vi "超标留样启动流程.vi"   [LabVIEW 2016, in "超标留样集成.lvlib" / "德润DR803L超标留样.lvlib"]
types:
  T1 = enum16{"open", "read", "write", "write single", "close"}
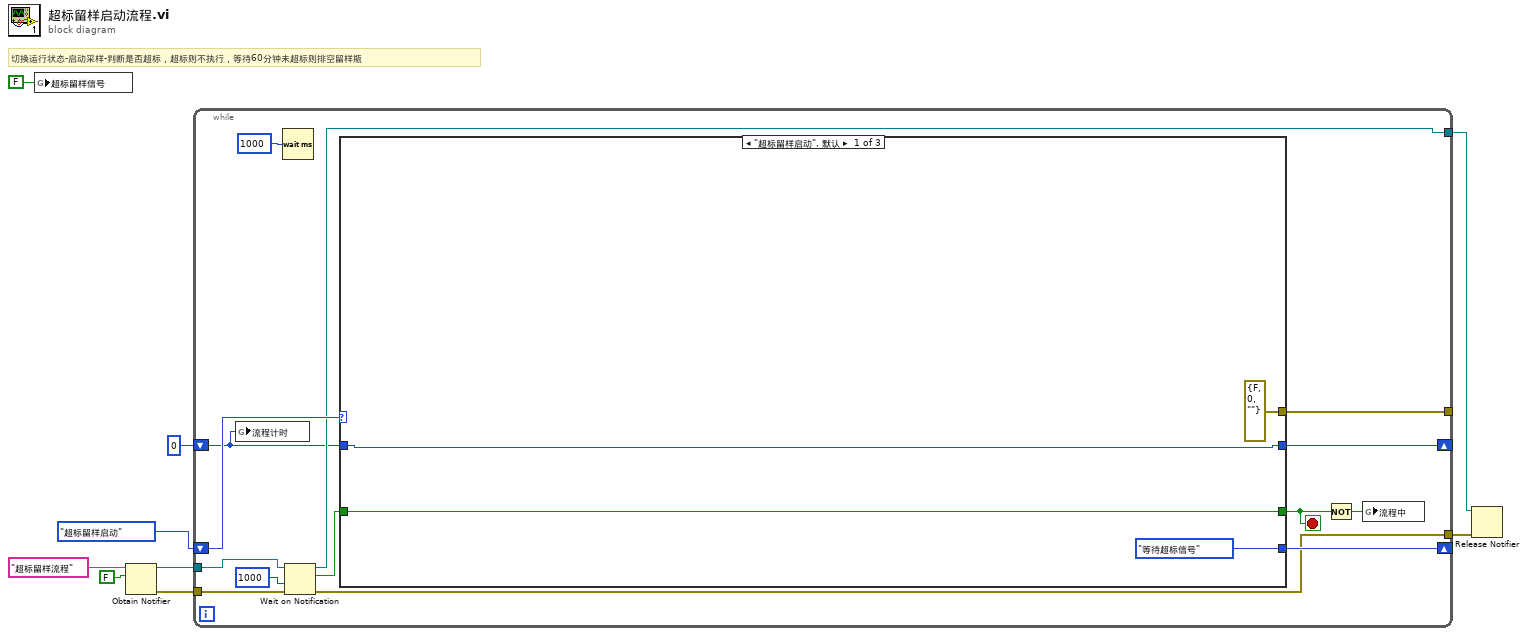
[diagram p0: block diagram]
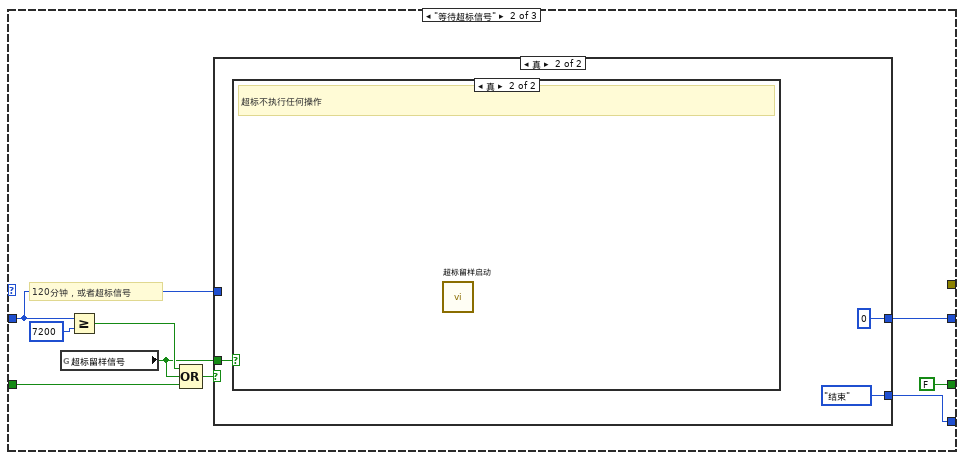
[diagram p2: hidden frame]
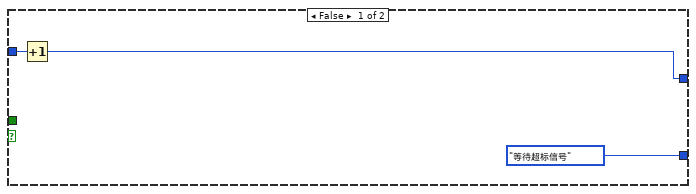
[diagram p3: hidden frame]
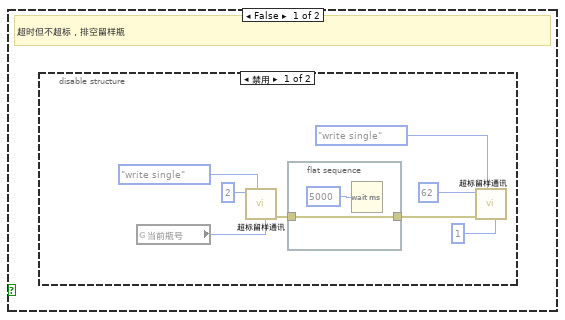
[diagram p4: hidden frame]
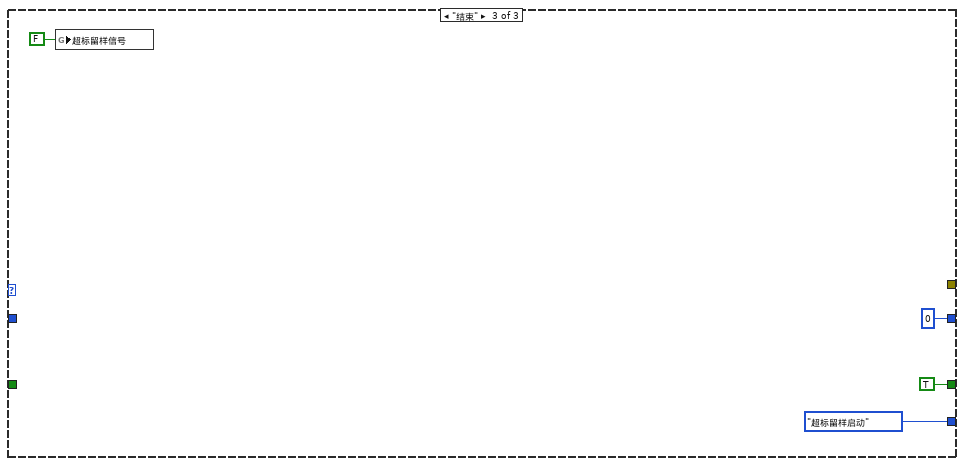
[diagram p6: hidden frame]
diagram:
  # "切换运行状态-启动采样-判断是否超标，超标则不执行，等待60分钟未超标则排空留样瓶"
  n1 = global write "串口参数断电保存全局变量.vi" "超标留样信号"(FALSE ("采样完成")) -> ()
  n2 = Obtain Notifier(name (unnamed)="超标留样流程" ("名称（未命名）"), notification data type=FALSE ("采样完成")) -> (notifier out=w5:refnum<notifier>, error out=w4:errorcluster)  [unwired: 2 in, 1 out]
  n3 = while {
    shift-right: [w17] -> _
    shift-left: enum16{"超标留样启动", "等待超标信号", "结束"}."超标留样启动" -> [w23]
    shift-right: [w21] -> _
    shift-left: 0 -> [w10]
    tunnel: w5 -> [w20]
    tunnel: w4 -> [w19]
    tunnel: [w15] -> _
    tunnel: [w12] -> w2
    tunnel: [w11] -> w1
    stop <- w13 stop-if-true
    n4 = global write "串口参数断电保存全局变量.vi" "流程计时"(w10) -> ()
    n5 = Wait (ms)(milliseconds to wait=u32 1000 ("等待时间（毫秒）")) -> ()  [unwired: 1 out]
    n6 = Wait on Notification(notifier=w20, timeout in ms (-1)=1000 ("超时毫秒(-1)"), error in (no error)=w19) -> (notifier out=w12:refnum<notifier>, notification=w14:bool, error out=w11:errorcluster)  [unwired: 1 in, 1 out]
    n7 = case shown="\"超标留样启动\", 默认" w23 {
      tunnel: w10 -> [w26 w32 _]
      tunnel: [w26 w34 0] -> w21
      tunnel: [enum16{"超标留样启动", "等待超标信号", "结束"}."等待超标信号" w31 enum16{"超标留样启动", "等待超标信号", "结束"}."超标留样启动"] -> w17
      tunnel: [w25 FALSE TRUE] -> w13
      tunnel: [errorcluster {"status"=FALSE, "code"=0, "source"=""} ("error out") _ _] -> w15
      tunnel: w14 -> [w25 w28 _]
      frame "超标留样启动", Default {
      }
      frame "等待超标信号" {
        # "120分钟，或者超标信号"
        n8 = global read "串口参数断电保存全局变量.vi" "超标留样信号"() -> (w29:bool)
        n9 = Greater Or Equal?(x=w32, y=7200) -> (x >= y?=w35:bool)
        n10 = Compound Arithmetic op=OR ("复合运算")(w35, w29, w28) -> (w33:bool)
        n11 = case shown="真" w33 {
          tunnel: [enum16{"超标留样启动", "等待超标信号", "结束"}."等待超标信号" enum16{"超标留样启动", "等待超标信号", "结束"}."结束"] -> w31
          tunnel: w32 -> [w39 _]
          tunnel: [w38 0] -> w34
          tunnel: w29 -> [_ w40]
          frame False {
            n12 = Increment(x=w39) -> (x+1=w38:i32)
          }
          frame True {
            n13 = case shown="真" w40 {
              frame False {
                # "超时但不超标，排空留样瓶"
                n14 = disable-structure shown="禁用" {
                  frame Disabled {
                    n15 = global read "超标留样全局.vi" "当前瓶号"() -> (w43:u16)
                    n16 = call "超标留样通讯.vi"("value"=w43, "STEP"=T1."write single", "starting address"=2 ("索引")) -> ("error out"=w49:errorcluster)  [unwired: 6 in, 2 out]
                    n17 = flat-sequence {
                      tunnel: w49 -> [w51]
                      tunnel: [w51] -> w50
                      frame #0 {
                        n18 = Wait (ms)(milliseconds to wait=u32 5000 ("等待时间（毫秒）")) -> ()  [unwired: 1 out]
                      }
                    }
                    n19 = call "超标留样通讯.vi"("value"=u16 1 ("新元素/子数组"), "STEP"=T1."write single", "Error in"=w50, "starting address"=62 ("索引")) -> ()  [unwired: 5 in, 3 out]
                  }
                  frame Enabled {
                  }
                }
              }
              frame True {
                # "超标不执行任何操作"
                n20 = call "超标留样启动.vi"() -> ()  [unwired: 11 in, 1 out]
              }
            }
          }
        }
      }
      frame "结束" {
        n21 = global write "串口参数断电保存全局变量.vi" "超标留样信号"(FALSE ("采样完成")) -> ()
      }
    }
    n22 = Not(x=w13) -> (.not. x?=w16:bool)
    n23 = global write "串口参数断电保存全局变量.vi" "流程中"(w16) -> ()
  }
  n24 = Release Notifier(notifier=w2, error in (no error)=w1) -> ()  [unwired: 1 in, 3 out]
